vi "Configure DAQ AI.vi"(8 "error in":errorcluster, 10 "Task Name":string, 11 "DAQ Configuration":T1 {"Terminal Config" items=["Default"=-1, "RSE"=10083, "NRSE"=10078, "Differential"=10106, "Pseudodifferential"=12529]; "Min (V)" format="%#_13g"; "Max (V)" format="%#_13g"; "Sample Rate (Hz)" format="%#_13g"}) -> (0 "error out":errorcluster, 3 "DAQ Task ref out":refnum<k21>)   [LabVIEW 2021, in "XNET-CAN-Signal-Logger.lvlib"]
uses:
  XNET-CAN-Signal-Logger.lvlib
  Typedef/Def-DAQ AI Configuration.ctl
  <vilib>/DAQmx/create/channels.llb/DAQmx Create Channel (AI-Voltage-Basic).vi
  <vilib>/DAQmx/configure/timing.llb/DAQmx Timing (Sample Clock).vi
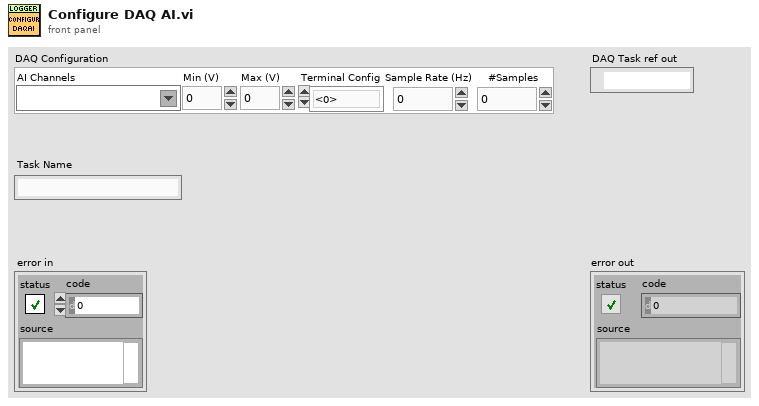
[diagram p1: front panel]
types:
  T1 = typedef "XNET-CAN-Signal-Logger.lvlib/Def-DAQ AI Configuration.ctl" = cluster{"AI Channels":tag, "Min (V)":dbl, "Max (V)":dbl, "Terminal Config":i32, "Sample Rate (Hz)":dbl, "#Samples":i32}
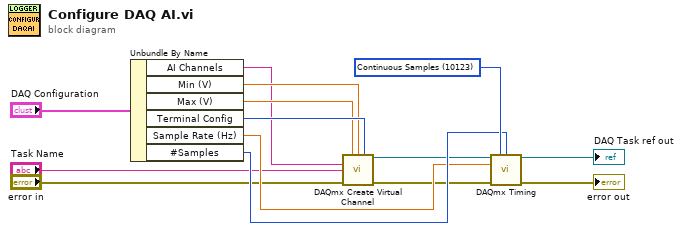
[diagram p0: block diagram]
diagram:
  w14 = 10123 items=["Finite Samples"=10178, "Continuous Samples"=10123, "Hardware Timed Single Point"=12522] ("sample mode")
  n1 = Unbundle By Name("DAQ Configuration") -> ("AI Channels"=w2:tag, "Min (V)"=w10:dbl, "Max (V)"=w9:dbl, "Terminal Config"=w11:i32, "Sample Rate (Hz)"=w12:dbl, "#Samples"=w13:i32)
  n2 = call-poly <vilib>:"DAQmx Create Virtual Channel.vi"("maximum value"=w9, "minimum value"=w10, "input terminal configuration"=w11, "physical channels"=w2, "name to assign"="Task Name", "error in"="error in") -> ("task out"=w6:refnum<k21>, "error out"=w5:errorcluster)  [unwired: 8 in]
  n3 = call-poly <vilib>:"DAQmx Timing.vi"("task/channels in"=w6, "sample mode"=w14, "samples per channel"=w13, "rate"=w12, "error in"=w5) -> ("task out"=→"DAQ Task ref out":refnum<k21>, "error out"=→"error out":errorcluster)  [unwired: 9 in]
